vi "SetComparisonType.vi"(8 "error in":errorcluster, 10 "ComparisonType":T1, 11 "RealMeasureLimit in":refnum<class "RealMeasureLimit.lvclass">) -> (0 "error out":errorcluster, 3 "RealMeasureLimit out":refnum<class "RealMeasureLimit.lvclass">)   [LabVIEW 2021, in "ProligentXMLGenerator.lvlib" / "RealMeasureLimit.lvclass"]
doc: "Real Measure Limit Comparison Type"
uses:
  RealMeasureLimit.lvclass
  RealMeasureLimit.lvclass/RealMeasureLimit.ctl
  RangeMeasureLimit/RangeMeasureLimit.lvclass
  Base/Decimal/Decimal.lvclass
  RangeMeasureLimit/ComparisonType.ctl
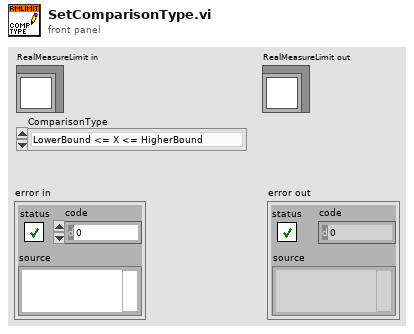
[diagram p1: front panel]
types:
  T1 = typedef "ProligentXMLGenerator.lvlib/RangeMeasureLimit.lvclass/ComparisonType.ctl" = enum16{"LowerBound <= X <= HigherBound", "LowerBound < X <= HigherBound", "LowerBound <= X < HigherBound", "LowerBound < X < HigherBound", "LowerBound <= X", "LowerBound < X", "X <= HigherBound", "X < HigherBound", "X == HigherBound", "X != HigherBound", "X <= LowerBound OR HigherBound <= X", "X < LowerBound OR HigherBound <= X", "X <= LowerBound OR HigherBound < X", "X < LowerBound OR HigherBound < X"}
  T2 = typedef "ProligentXMLGenerator.lvlib/RealMeasureLimit.lvclass/Data.ctl" = cluster{"LowerBound":refnum<class "Decimal.lvclass">, "HigherBound":refnum<class "Decimal.lvclass">}
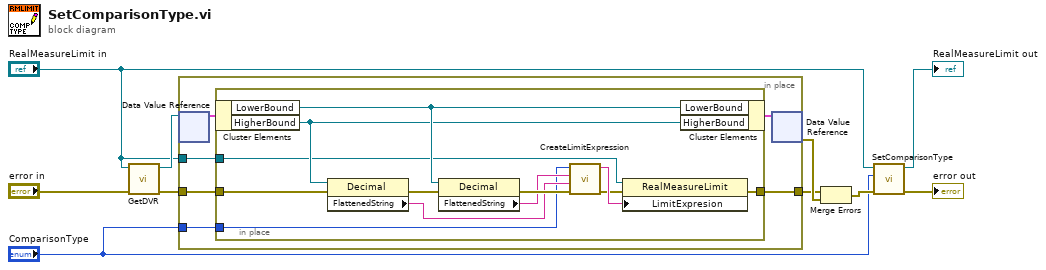
[diagram p0: block diagram]
diagram:
  n1 = call "GetDVR.vi"("error in"="error in", "RealMeasureLimit"="RealMeasureLimit in") -> ("error out"=w8:errorcluster, "DVRReference"=w9:refnum<data-value>)  [unwired: 8 in]
  n2 = in-place "In Place Element Structure" {
    in-place-border: "ComparisonType" -> [w16]
    in-place-border: w8 -> [w13]
    in-place-border: "RealMeasureLimit in" -> [w12]
    in-place-border: [w11] -> w6
    n3 = in-place-dvr #1(w9) -> (w15:T2)  [unwired: 1 out]
    n4 = in-place "In Place Element Structure" {
      in-place-border: w16 -> [w19]
      in-place-border: w13 -> [w28]
      in-place-border: w12 -> [w18]
      in-place-border: [w17] -> w11
      n5 = in-place-cluster #2(w15) -> ("LowerBound"=w21:refnum<class "Decimal.lvclass">, "HigherBound"=w20:refnum<class "Decimal.lvclass">)
      n6 = property class="Decimal"(reference=w20, error in=w28) -> (error out=w25:errorcluster, "FlattenedString"=w23:string)  [unwired: 1 out]
      n7 = property class="Decimal"(reference=w21, error in=w25) -> (error out=w24:errorcluster, "FlattenedString"=w22:string)  [unwired: 1 out]
      n8 = call "CreateLimitExpression.vi"("error in"=w24, "HigherBound"=w23, "LowerBound"=w22, "ComparisonType"=w19) -> ("error out"=w26:errorcluster, "LimitExpression"=w27:string)  [unwired: 6 in]
      n9 = property class="RealMeasureLimit"(reference=w18, error in=w26, "LimitExpresion"=w27) -> (error out=w17:errorcluster)  [unwired: 1 out]
      n10 = in-place-cluster #2("LowerBound"=w21, "HigherBound"=w20) -> (w14:T2)
    }
    n11 = in-place-dvr #1(w14) -> (w7:errorcluster)  [unwired: 1 out]
  }
  n12 = Merge Errors(w6, w7) -> (w4:errorcluster)
  n13 = call-parent "SetComparisonType.vi"("error in"=w4, "ComparisonType"="ComparisonType", "RangeMeasureLimit in"="RealMeasureLimit in") -> ("error out"=→"error out":errorcluster, "RangeMeasureLimit out"=→"RealMeasureLimit out":refnum<class "RealMeasureLimit.lvclass">)  [unwired: 7 in]
